vi "View TDMS Chan.vi"() -> ()   [LabVIEW 2024]
panel:
  out "Waveform Graph":waveform(i16)(graph)
  in  "count (-1: all)":i64=-1 format="%d (x%x)"
  in  "offset (0)":i64 format="%d (x%x)"
  in  "channel":string="in0"
  in  "group":string="p"
  in  "Defragment":bool
  in  "file path":path
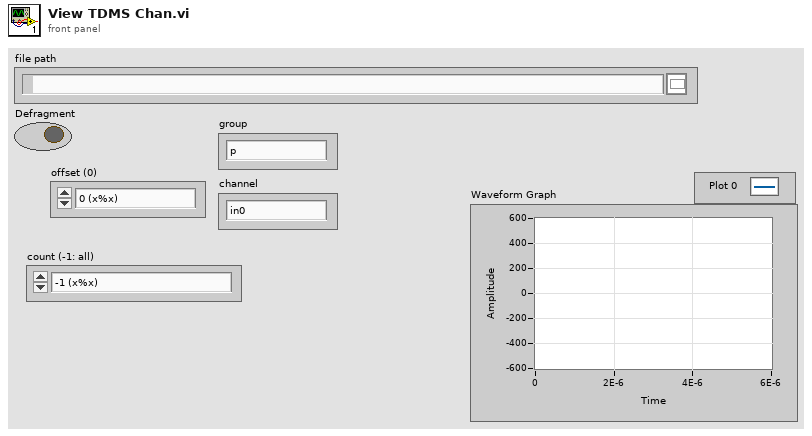
[diagram p1: front panel]
types:
  T1 = enum16{"open", "open or create", "create or replace", "create", "open (read-only)"}
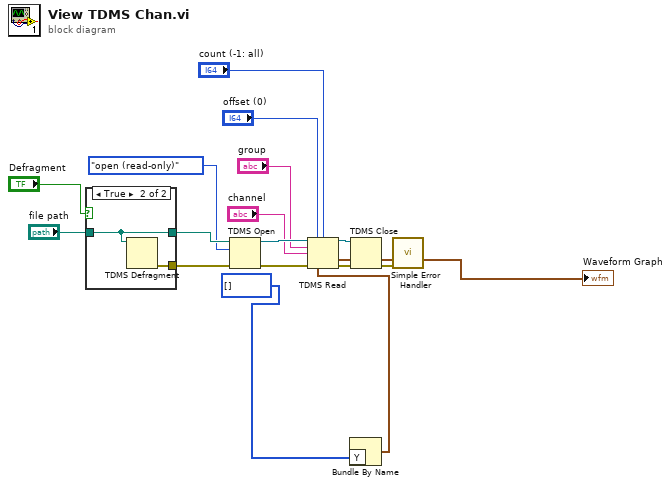
[diagram p0: block diagram]
diagram:
  n1 = case shown="True" "Defragment" {
    tunnel: "file path" -> [w18 w19]
    tunnel: [_ w20] -> w15
    tunnel: [w18 w19] -> w14
    frame False {
    }
    frame True {
      n2 = TDMS Defragment(7:w19) -> (0:w20:errorcluster)  [unwired: 1 in]
    }
  }
  n3 = TDMS Open(8:w15, 10:T1."open (read-only)" ("operation (0:open)"), 11:w14) -> (0:w7:errorcluster, 3:w12:refnum<k34>)  [unwired: 4 in]
  n4 = Bundle By Name("Y"=i16[] []) -> (w2:waveform(i16))  [unwired: 1 in]
  n5 = TDMS Read(0:w12, 1:"offset (0)", 2:"count (-1: all)", 5:"group", 7:"channel", 11:w7, 12:w2) -> (4:w8:refnum<k34>, 10:→"Waveform Graph":waveform(i16), 15:w9:errorcluster)  [unwired: 1 in, 3 out]
  n6 = TDMS Close(8:w9, 11:w8) -> (0:w6:errorcluster)  [unwired: 1 out]
  n7 = call <vilib>:"Simple Error Handler.vi"("error in (no error)"=w6) -> ()  [unwired: 4 in, 5 out]
